vi "Mcp2210 Get Last Error.vi"(8 "error in (no error)":errorcluster) -> (0 "error out":errorcluster, 3 "function return":i32(ring) items=["E_SUCCESS"=0, "E_ERR_UNKOWN_ERROR"=-1, "E_ERR_INVALID_PARAMETER"=-2, "E_ERR_NULL"=-10, "E_ERR_MALLOC"=-20, "E_ERR_INVALID_HANDLE_VALUE"=-30, "E_ERR_FIND_DEV"=-100, "E_ERR_NO_SUCH_INDEX"=-101, "E_ERR_DEVICE_NOT_FOUND"=-103, "E_ERR_INTERNAL_BUFFER_TOO_SMALL"=-104, "E_ERR_OPEN_DEVICE_ERROR"=-105, "E_ERR_CONNECTION_ALREADY_OPENED"=-106, "E_ERR_CLOSE_FAILED"=-107, "E_ERR_NO_SUCH_SERIALNR"=-108, "E_ERR_HID_RW_TIMEOUT"=-110, "E_ERR_HID_RW_FILEIO"=-111, "E_ERR_CMD_FAILED"=-200, "E_ERR_CMD_ECHO"=-201, "E_ERR_SUBCMD_ECHO"=-202, "E_ERR_SPI_CFG_ABORT"=-203, "E_ERR_SPI_EXTERN_MASTER"=-204, "E_ERR_SPI_TIMEOUT"=-205, "E_ERR_SPI_RX_INCOMPLETE"=-206, "E_ERR_SPI_XFER_ONGOING"=-207, "E_ERR_BLOCKED_ACCESS"=-300, "E_ERR_EEPROM_WRITE_FAIL"=-301, "E_ERR_NVRAM_LOCKED"=-350, "E_ERR_WRONG_PASSWD"=-351, "E_ERR_ACCESS_DENIED"=-352, "E_ERR_NVRAM_PROTECTED"=-353, "E_ERR_PASSWD_CHANGE"=-354, "E_ERR_STRING_DESCRIPTOR"=-400, "E_ERR_STRING_TOO_LARGE"=-401])   [LabVIEW 2015, in "mcp2210.lvlib"]
doc: "Returns the detailed error code of the last library function call whose prototype is\nnot making this possible. The library functions that need this support are:\n- M_Mcp2210_OpenByIndex()\n- M_Mcp2210_OpenBySN()\n!!! Important note !!!\nIn order to avoid the last error code being altered by other API calls, please make sure that\nM_Mcp2210_GetLastError() is called immediately after the API listed above and save the returned value\naccordingly.\nParameters:\nInputs:\n- none\nOutputs:\n- none\nReturns:\n- M_E_SUCCESS or negative error code: please see the description of the above listed API calls\n\nMCP2210_DLL_UM_API int __stdcall Mcp2210_GetLastError();"
uses:
  <userlib>/mcp2210/mcp2210.lvlib
  <userlib>/mcp2210/mcp2210_dll_um_x86.dll
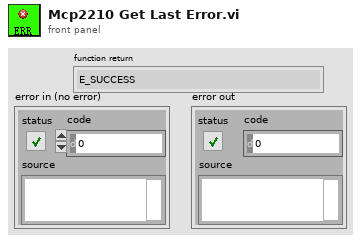
[diagram p1: front panel]
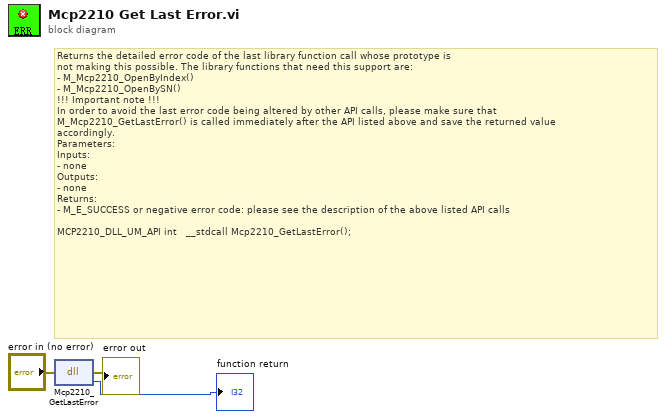
[diagram p0: block diagram]
diagram:
  # "Returns the detailed error code of the last library function call whose prototype is\nnot making this possible. The library functions that need this support are:\n- M_Mcp2210_OpenByIndex()\n- M_Mcp2210_OpenBySN()\n!!! Important note !!!\nIn order to avoid the last error code being altered by other API calls, please make sure that\nM_Mcp2210_GetLastError() is called immediately after the API listed above and save the returned value\naccordingly.\nParameters:\nInputs:\n- none\nOutputs:\n- none\nReturns:\n- M_E_SUCCESS or negative error code: please see the description of the above listed API calls\n\nMCP2210_DLL_UM_API int   __stdcall Mcp2210_GetLastError();"
  n1 = dll-call lib="D:/LabVIEW 2015/user.lib/mcp2210/mcp2210_dll_um_x86.*" fn="Mcp2210_GetLastError"(error in="error in (no error)") -> (error out=→"error out":errorcluster, →"function return":i32)  [unwired: 2 in, 1 out]
